vi "Pockels power to volts.vi"(11 "Pockels power (%)":dbl) -> (1 "Back-aperture power (mW)":dbl, 2 "Power after the objective (mW)":dbl, 3 "Pockels control voltage (V)":dbl)   [LabVIEW 2013]
uses:
  Typedefs/Functional global standard states.ctl
  Configuration code/Calibration/Globals/gl_Calibration globals.vi
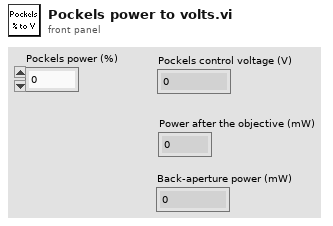
[diagram p1: front panel]
types:
  T1 = typedef "Functional global standard states.ctl" = enum16{"Initialise", "Read", "Write", "Load", "Save", "Clear"}
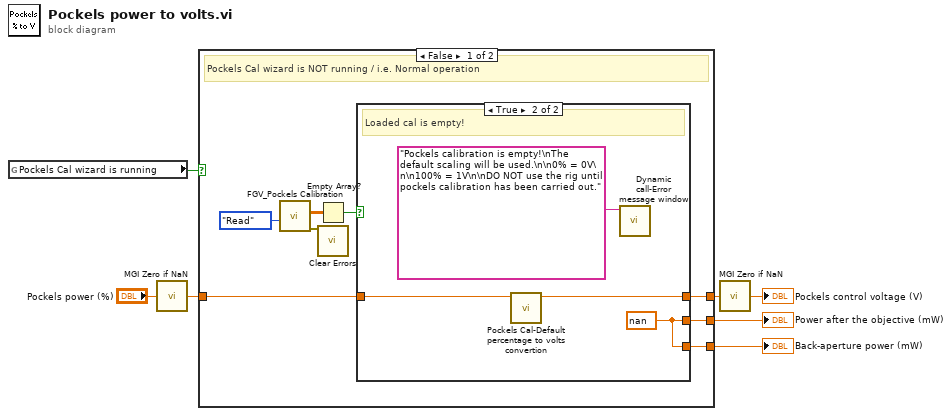
[diagram p0: block diagram]
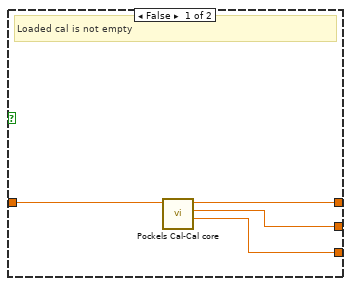
[diagram p2: hidden frame]
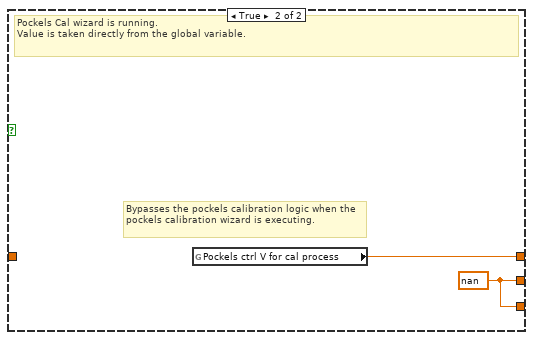
[diagram p3: hidden frame]
diagram:
  n1 = global read "gl_Calibration globals.vi" "Pockels Cal wizard is running"() -> (w7:bool)
  n2 = call "MGI Zero if NaN.vi"("Number In"="Pockels power (%)") -> ("Number Out"=w1:dbl)
  n3 = case shown="False" w7 {
    tunnel: [w15 w25] -> w3
    tunnel: w1 -> [w14 _]
    tunnel: [w10 w24] -> w6
    tunnel: [w9 w24] -> w5
    frame False {
      # "Pockels Cal wizard is NOT running / i.e. Normal operation"
      n4 = call "FGV_Pockels Calibration.vi"("Function"=Functional_global_standard_states."Read") -> ("error out"=w8:errorcluster, "Pockels calibration data (Single wavelength)"=w12:dbl[][])  [unwired: 4 in, 5 out]
      n5 = Empty Array?(array=w12) -> (empty?=w11:bool)
      n6 = call <vilib>:"Clear Errors.vi"("error in (no error)"=w8) -> ()  [unwired: 6 in, 1 out]
      n7 = case shown="True" w11 {
        tunnel: [w18 w21] -> w15
        tunnel: w14 -> [w19 w22]
        tunnel: [w17 w20] -> w10
        tunnel: [w16 w20] -> w9
        frame False {
          # "Loaded cal is not empty"
          n8 = call "Pockels Cal-Cal core.vi"("Pockels power (%)"=w19) -> ("Back-aperture power (mW)"=w17:dbl, "Power after the objective (mW)"=w16:dbl, "Pockels Volts"=w18:dbl)  [unwired: 8 in]
        }
        frame True {
          w20 = nan ("Normalised power (mW)")
          # "Loaded cal is empty!"
          n9 = call "Pockels Cal-Default percentage to volts convertion.vi"("Pockels power"=w22) -> ("Pockels Volts"=w21:dbl)  [unwired: 10 in]
          n10 = call "Dynamic call-Error message window.vi"("Error Message"="Pockels calibration is empty!\nThe default scaling will be used.\n\n0% = 0V\n\n100% = 1V\n\nDO NOT use the rig until pockels calibration has been carried out.") -> ()  [unwired: 10 in, 1 out]
        }
      }
    }
    frame True {
      w24 = nan ("Normalised power (mW)")
      # "Bypasses the pockels calibration logic when the pockels calibration wizard is executing."
      # "Pockels Cal wizard is running.\nValue is taken directly from the global variable."
      n11 = global read "gl_Calibration globals.vi" "Pockels ctrl V for cal process"() -> (w25:dbl)
    }
  }
  "Back-aperture power (mW)" <- w6
  "Power after the objective (mW)" <- w5
  n12 = call "MGI Zero if NaN.vi"("Number In"=w3) -> ("Number Out"=→"Pockels control voltage (V)":dbl)
